vi "AM Initialize Points.vi"(8 "error in (no error)":errorcluster, 10 "Message Data":variant, 11 "Hardware Resources in":T1) -> (0 "error out":errorcluster, 3 "Hardware Resources out":T1)   [LabVIEW 2020, in "Motion.lvlib"]
doc: "Initialize the hardware references."
uses:
  Motion.lvlib
  AM Configuration.ctl
  support/Message Queue/Message Cluster.ctl
  support/Message Queue/Message Queue.lvlib
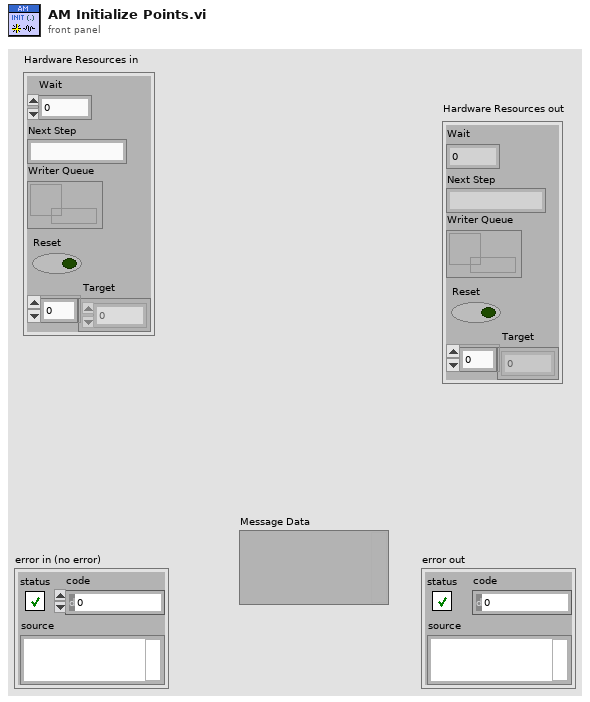
[diagram p1: front panel]
types:
  T1 = typedef "Motion.lvlib/AM Configuration.ctl" = cluster{"Wait":dbl, "Next Step":string, "Writer Queue":refnum<queue>, "Reset":bool, "Target":dbl[]}
  T2 = cluster{"Temperature":dbl[], "wait":dbl, "Step":u8, "Current":dbl[], "Strirrer":dbl[], "PS delay":dbl, "PS Stop":dbl, "Volt":dbl[]}
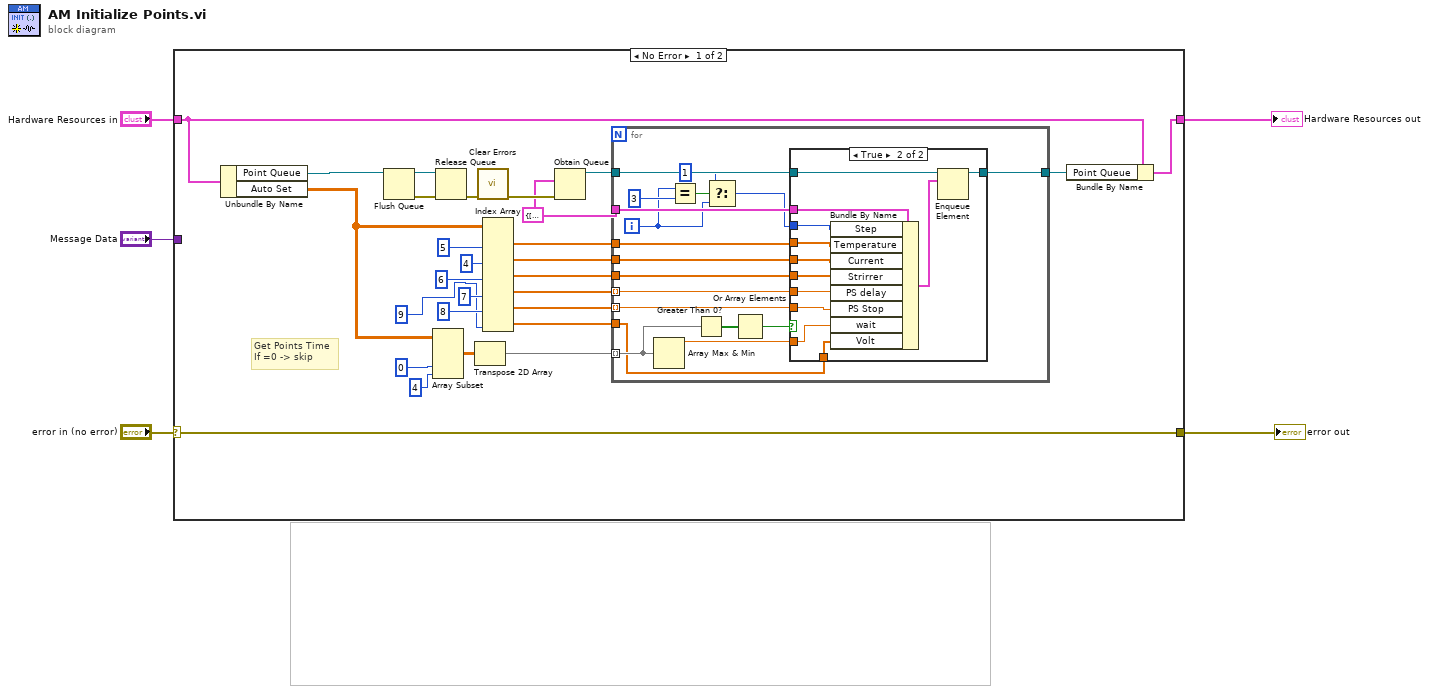
[diagram p0: block diagram]
diagram:
  n1 = case shown="No Error" "error in (no error)" {
    selector: "error in (no error)" -> [w31 w65]
    tunnel: [w31 w65] -> w4
    tunnel: "Hardware Resources in" -> [w32 w66]
    tunnel: [w33 w66] -> w1
    tunnel: "Message Data" -> [_ _]
    frame No Error {
      w26 = T2 {"Temperature"=[], "wait"=0.0, "Step"=0, "Current"=[], "Strirrer"=[], "PS delay"=0.0, "PS Stop"=0.0, "Volt"=[]}
      # "Get Points Time\nIf =0 -> skip"
      n2 = Unbundle By Name(w32) -> ("Point Queue"=w28:refnum<queue>, "Auto Set"=w18:dbl[][])
      n3 = Flush Queue(queue=w28) -> (queue out=w24:refnum<queue>, error out=w25:errorcluster)  [unwired: 1 in, 1 out]
      n4 = Array Subset(array=w18, index (col)=0 ("index"), length (col)=4 ("length")) -> (w20:dbl[][])  [unwired: 2 in]
      n5 = Release Queue(queue=w24, error in (no error)=w25) -> (error out=w23:errorcluster)  [unwired: 1 in, 2 out]
      n6 = Transpose 2D Array(2D array=w20) -> (transposed array=w19:dbl[][])
      n7 = call <vilib>:"Clear Errors.vi"("error in (no error)"=w23) -> ("error out"=w29:errorcluster)  [unwired: 5 in, 1 out]
      n8 = Index Array(array=w18, index (col) #1=5 ("disabled index (col)"), index (col) #2=4 ("index (col)"), index (col) #3=6 ("index (col)"), index (col) #4=7 ("index (col)"), index (col) #5=8 ("index (col)"), index (col) #6=9 ("index (col)")) -> (element #1=w16:dbl[], element #2=w14:dbl[], element #3=w12:dbl[], element #4=w6:dbl[], element #5=w9:dbl[], element #6=w7:dbl[])  [unwired: 6 in]
      n9 = Obtain Queue(element data type=w26, error in (no error)=w29) -> (queue out=w27:refnum<queue>)  [unwired: 3 in, 2 out]
      n10 = for {
        tunnel: w27 -> [w50]
        tunnel: [w51] -> w30
        tunnel: w26 -> [w49]
        tunnel: w19 -> [w46] mode=indexing
        tunnel: w16 -> [w44]
        tunnel: w14 -> [w43]
        tunnel: w12 -> [w42]
        tunnel: w6 -> [w36] mode=indexing
        tunnel: w9 -> [w35] mode=indexing
        tunnel: w7 -> [w34]
        i -> [w39]
        n11 = Array Max & Min(array=w46) -> (max value=w45:dbl)  [unwired: 3 out]
        n12 = Equal?(x=w39, y=3) -> (x = y?=w40:bool)
        n13 = Greater Than 0?(x=w46) -> (x > 0?=w48:bool[])
        n14 = Select(t=1, s=w40, f=w39) -> (s? t:f=w38:i32)
        n15 = Or Array Elements(Boolean array=w48) -> (logical OR=w47:bool)
        n16 = case shown="True" w47 {
          tunnel: [w52 w64] -> w51
          tunnel: w50 -> [w52 w63]
          tunnel: w49 -> [_ w61]
          tunnel: w38 -> [_ w57]
          tunnel: w45 -> [_ w56]
          tunnel: w44 -> [_ w60]
          tunnel: w43 -> [_ w59]
          tunnel: w42 -> [_ w58]
          tunnel: w36 -> [_ w55]
          tunnel: w35 -> [_ w54]
          tunnel: w34 -> [_ w53]
          frame False {
          }
          frame True {
            n17 = Bundle By Name(cluster=w61, "Step"=w57, "Temperature"=w60, "Current"=w59, "Strirrer"=w58, "PS delay"=w55, "PS Stop"=w54, "wait"=w56, "Volt"=w53) -> (w62:T2)
            n18 = Enqueue Element(queue=w63, element=w62) -> (queue out=w64:refnum<queue>)  [unwired: 2 in, 2 out]
          }
        }
      }
      n19 = Bundle By Name(cluster=w32, "Point Queue"=w30) -> (w33:T1)
    }
    frame Error {
    }
  }
  "Hardware Resources out" <- w1
  "error out" <- w4
